vi "Output current I (SubVI).vi"(0 "I_1":dbl, 1 "R_s":dbl, 2 "V":dbl, 5 "I_ph":dbl, 7 "N_s":dbl, 9 "I_sh":dbl, 12 "T":dbl, 13 "n":dbl, 14 "I_0":dbl) -> (4 "I":dbl)   [LabVIEW 2024]
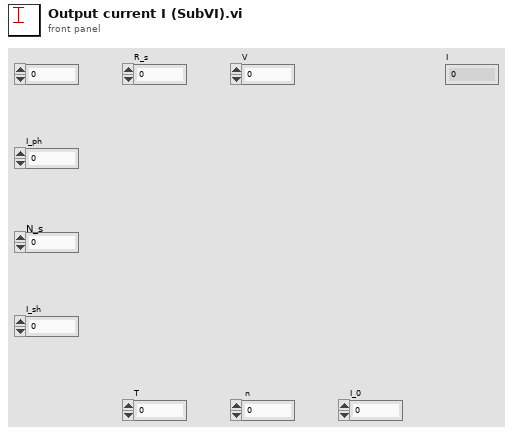
[diagram p1: front panel]
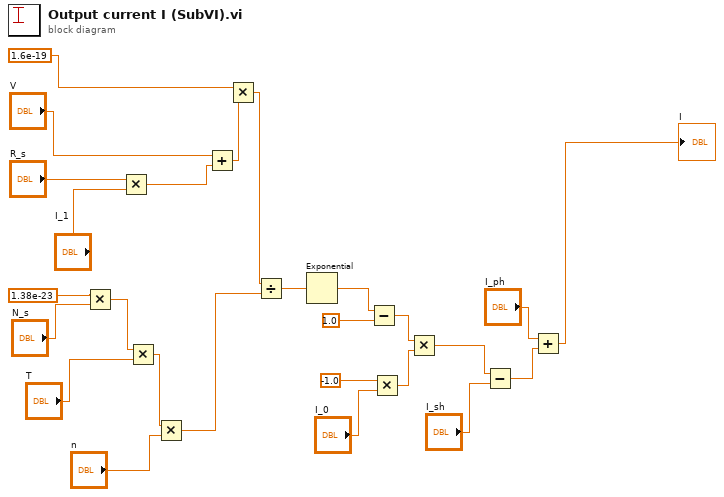
[diagram p0: block diagram]
diagram:
  n1 = Multiply(x=1.38e-23, y="N_s") -> (x*y=w22:dbl)
  n2 = Multiply(x="R_s", y="I_1") -> (x*y=w15:dbl)
  n3 = Multiply(x=w22, y="T") -> (x*y=w19:dbl)
  n4 = Multiply(x=w19, y="n") -> (x*y=w18:dbl)
  n5 = Add(x="V", y=w15) -> (x+y=w14:dbl)
  n6 = Multiply(x=1.6e-19, y=w14) -> (x*y=w12:dbl)
  n7 = Divide(x=w12, y=w18) -> (x/y=w4:dbl)
  n8 = Exponential(1:w4) -> (0:w2:dbl)
  n9 = Subtract(x=w2, y=1.0) -> (x-y=w1:dbl)
  n10 = Multiply(x=-1.0, y="I_0") -> (x*y=w9:dbl)
  n11 = Multiply(x=w1, y=w9) -> (x*y=w8:dbl)
  n12 = Subtract(x=w8, y="I_sh") -> (x-y=w6:dbl)
  n13 = Add(x="I_ph", y=w6) -> (x+y=→"I":dbl)
